vi "AddActiveSubscription.vi"(0 "STOMP in":refnum<class "STOMP.lvclass">, 2 "activeSubscription":T1, 5 "error in (no error)":errorcluster) -> (14 "STOMP out":refnum<class "STOMP.lvclass">, 19 "error out":errorcluster)   [LabVIEW 2017, in "LabVIEW STOMP.lvlib" / "STOMP.lvclass"]
uses:
  STOMP.lvclass
  Typedefs/Type_ActiveSubscription.ctl
  Typedefs/Type_AckHeader.ctl
  Typedefs/Type_FrameHeader.ctl
  STOMP.lvclass/STOMP.ctl
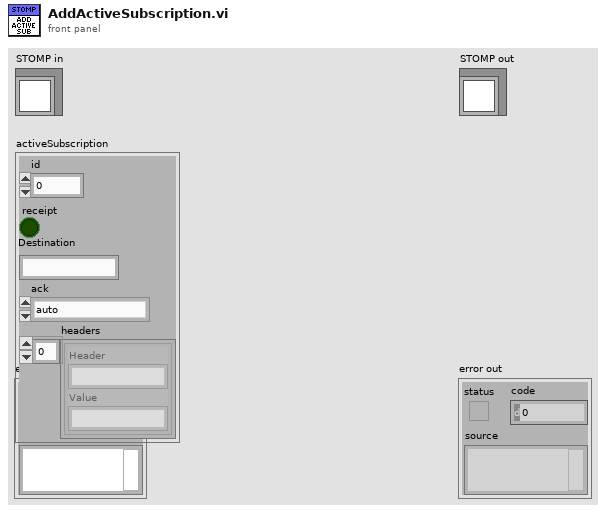
[diagram p1: front panel]
types:
  T1 = typedef "LabVIEW STOMP.lvlib/STOMP.lvclass/Type_ActiveSubscription.ctl" = cluster{"id":u64, "receipt":bool, "Destination":string, "ack":T2, "headers":T3[]}
  T2 = typedef "LabVIEW STOMP.lvlib/STOMP.lvclass/Type_AckHeader.ctl" = enum16{"auto", "client", "client-individual"}
  T3 = typedef "LabVIEW STOMP.lvlib/STOMP.lvclass/Type_FrameHeader.ctl" = cluster{"Header":string, "Value":string}
  T4 = typedef "LabVIEW STOMP.lvlib/STOMP.lvclass/ObjectAttributes.ctl" = cluster{"address":string, "port":u16, "ConnectionRef":refnum<k5>, "messageQueue":refnum<queue>, "receiptQueue":refnum<queue>, "errorQueue":refnum<queue>, "sendQueue":refnum<queue>, "currentReceiptNumber":u64, "currentSubscriptionId":u64, "closeConnection":bool, "activeSubscriptions":T5[]}
  T5 = typedef "Type_ActiveSubscription.ctl" = cluster{"id":u64, "receipt":bool, "Destination":string, "ack":T6, "headers":T3[]}
  T6 = typedef "Type_AckHeader.ctl" = enum16{"auto", "client", "client-individual"}
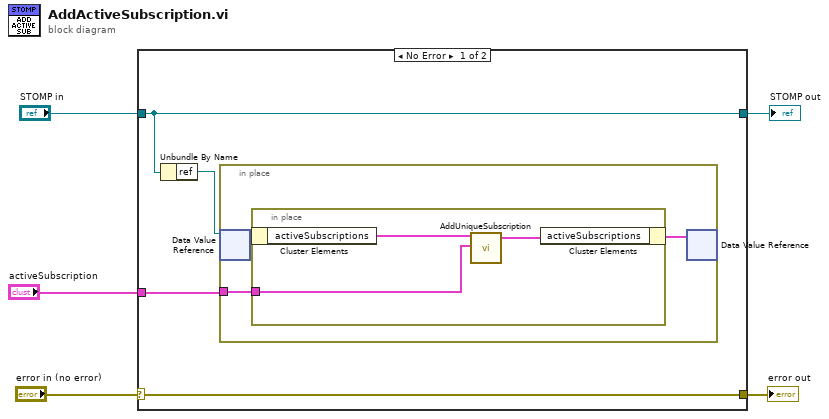
[diagram p0: block diagram]
diagram:
  n1 = case shown="No Error" "error in (no error)" {
    selector: "error in (no error)" -> [w9 w17]
    tunnel: [w9 w17] -> w4
    tunnel: [w6 w16] -> w2
    tunnel: "STOMP in" -> [w6 w16]
    tunnel: "activeSubscription" -> [w8 _]
    frame No Error {
      n2 = Unbundle By Name(w6) -> ("ref"=w7:refnum<data-value>)
      n3 = in-place {
        in-place-border: w8 -> [w12]
        n4 = in-place-dvr #1(w7) -> (w11:T4)  [unwired: 1 out]
        n5 = in-place {
          in-place-border: w12 -> [w14]
          n6 = in-place-cluster #2(w11) -> ("activeSubscriptions"=w15:T5[])
          n7 = call "AddUniqueSubscription.vi"("activeSubscriptions"=w15, "subscription"=w14) -> ("activeSubscriptions"=w13:T1[])  [unwired: 17 in]
          n8 = in-place-cluster #2("activeSubscriptions"=w13) -> (w10:T4)
        }
        n9 = in-place-dvr #1(w10) -> ()  [unwired: 2 out]
      }
    }
    frame Error {
    }
  }
  "error out" <- w4
  "STOMP out" <- w2
